vi "Acc-Dec.vi"(2 "Acc Rate":dbl, 3 "Y-Input 2":dbl, 4 "Y-Input 1":dbl) -> (0 "Y-Output 2":dbl, 1 "Y-Output 1":dbl)   [LabVIEW 2012]
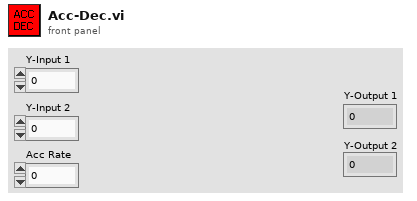
[diagram p1: front panel]
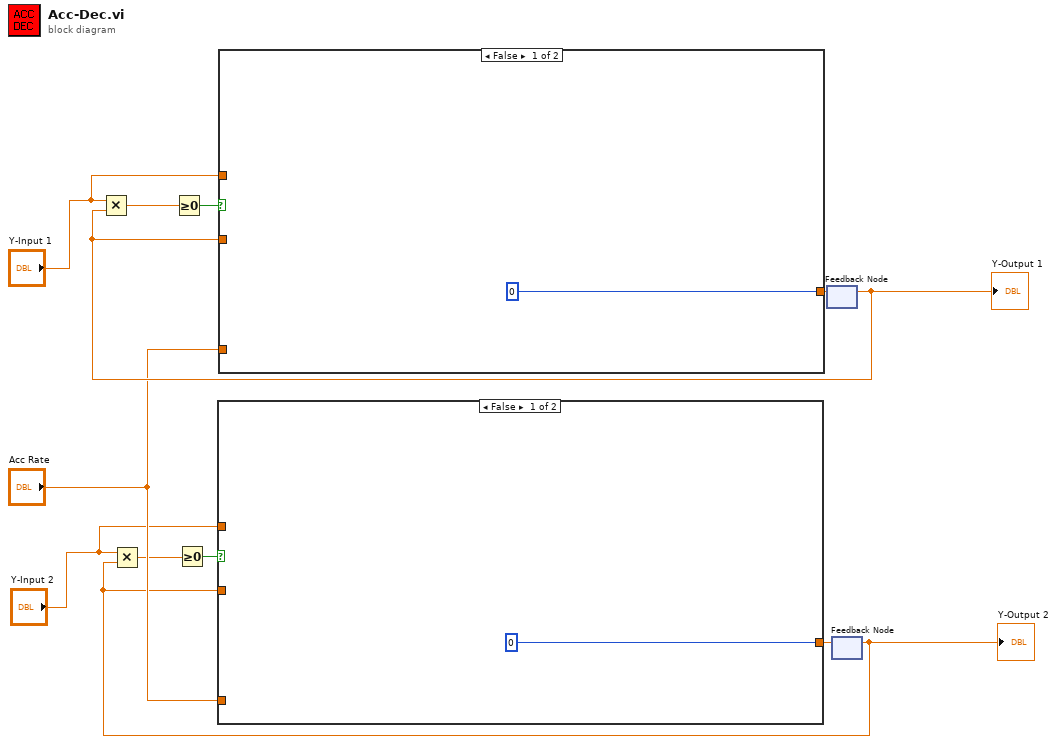
[diagram p0: block diagram]
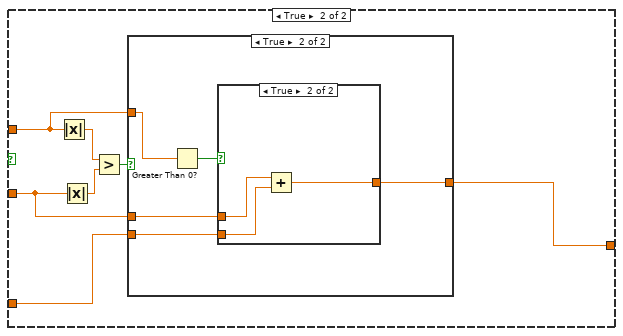
[diagram p2: hidden frame]
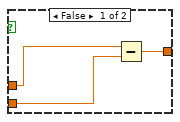
[diagram p4: hidden frame]
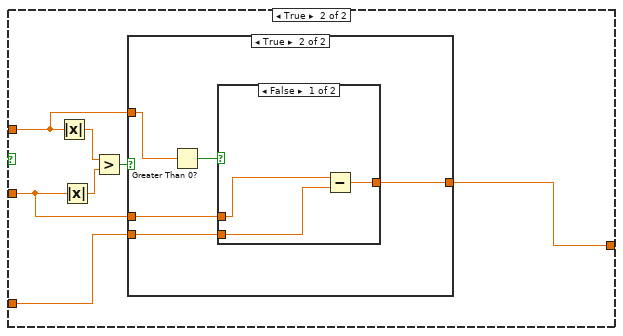
[diagram p5: hidden frame]
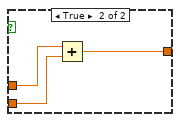
[diagram p7: hidden frame]
diagram:
  n1 = feedback #1() -> (w8:dbl)  [unwired: 1 in]
  "Y-Output 1" <- w8
  n2 = Multiply(x="Y-Input 1", y=w8) -> (x*y=w10:dbl)
  n3 = Greater Or Equal To 0?(x=w10) -> (x >= 0?=w11:bool)
  n4 = case shown="False" w11 {
    tunnel: [0 w16] -> w9
    tunnel: w8 -> [_ w13]
    tunnel: "Y-Input 1" -> [_ w15]
    tunnel: "Acc Rate" -> [_ w14]
    frame False {
    }
    frame True {
      n5 = Absolute Value(x=w15) -> (abs(x)=w19:dbl)
      n6 = Absolute Value(x=w13) -> (abs(x)=w18:dbl)
      n7 = Greater?(x=w19, y=w18) -> (0:w17:bool)
      n8 = case shown="True" w17 {
        tunnel: [w20 w21] -> w16
        tunnel: w15 -> [w20 w25]
        tunnel: w14 -> [_ w23]
        tunnel: w13 -> [_ w22]
        frame False {
        }
        frame True {
          n9 = Greater Than 0?(x=w25) -> (x > 0?=w24:bool)
          n10 = case shown="False" w24 {
            tunnel: w23 -> [w26 w31]
            tunnel: w22 -> [w27 w30]
            tunnel: [w28 w29] -> w21
            frame False {
              n11 = Subtract(x=w27, y=w26) -> (x-y=w28:dbl)
            }
            frame True {
              n12 = Add(x=w30, y=w31) -> (x+y=w29:dbl)
            }
          }
        }
      }
    }
  }
  n13 = feedback-in #1(w9) -> ()
  n14 = feedback #2() -> (w2:dbl)  [unwired: 1 in]
  "Y-Output 2" <- w2
  n15 = Multiply(x="Y-Input 2", y=w2) -> (x*y=w3:dbl)
  n16 = Greater Or Equal To 0?(x=w3) -> (x >= 0?=w5:bool)
  n17 = case shown="False" w5 {
    tunnel: [0 w36] -> w4
    tunnel: w2 -> [_ w33]
    tunnel: "Y-Input 2" -> [_ w35]
    tunnel: "Acc Rate" -> [_ w34]
    frame False {
    }
    frame True {
      n18 = Absolute Value(x=w35) -> (abs(x)=w39:dbl)
      n19 = Absolute Value(x=w33) -> (abs(x)=w38:dbl)
      n20 = Greater?(x=w39, y=w38) -> (0:w37:bool)
      n21 = case shown="True" w37 {
        tunnel: [w40 w41] -> w36
        tunnel: w35 -> [w40 w45]
        tunnel: w34 -> [_ w43]
        tunnel: w33 -> [_ w42]
        frame False {
        }
        frame True {
          n22 = Greater Than 0?(x=w45) -> (x > 0?=w44:bool)
          n23 = case shown="True" w44 {
            tunnel: w43 -> [w46 w51]
            tunnel: w42 -> [w47 w50]
            tunnel: [w48 w49] -> w41
            frame False {
              n24 = Subtract(x=w47, y=w46) -> (x-y=w48:dbl)
            }
            frame True {
              n25 = Add(x=w50, y=w51) -> (x+y=w49:dbl)
            }
          }
        }
      }
    }
  }
  n26 = feedback-in #2(w4) -> ()
